vi "USB2XXX_LINEX_MasterSchTest.vi"() -> ()   [LabVIEW 2010]
panel:
  in  "Get Sch":bool
  out "设置调度表成功？":bool
  in  "pInMsg 3":T1={"Timestamp"=50, "MsgType"=2, "CheckType"=0, "DataLen"=0, "Sync"=85, "PID"=3, "Data[0]"=0, "Data[1]"=0, "Data[2]"=0, "Data[3]"=0, "Data[4]"=0, "Data[5]"=0, "Data[6]"=0, "Data[7]"=0, "Check"=0, "Reserve"=0, "Reserve"=0} {"Sync" format="%x"; "PID" format="%x"; "Data[0]" format="%x"; "Data[1]" format="%x"; "Data[2]" format="%x"; "Data[3]" format="%x"; "Data[4]" format="%x"; "Data[5]" format="%x"; "Data[6]" format="%x"; "Data[7]" format="%x"; "Check" format="%x"; "Reserve" format="%x"; "Reserve" format="%x"}
  in  "pInMsg 2":T1={"Timestamp"=50, "MsgType"=1, "CheckType"=0, "DataLen"=8, "Sync"=85, "PID"=2, "Data[0]"=17, "Data[1]"=34, "Data[2]"=51, "Data[3]"=68, "Data[4]"=85, "Data[5]"=102, "Data[6]"=119, "Data[7]"=136, "Check"=0, "Reserve"=0, "Reserve"=0} {"Sync" format="%x"; "PID" format="%x"; "Data[0]" format="%x"; "Data[1]" format="%x"; "Data[2]" format="%x"; "Data[3]" format="%x"; "Data[4]" format="%x"; "Data[5]" format="%x"; "Data[6]" format="%x"; "Data[7]" format="%x"; "Check" format="%x"; "Reserve" format="%x"; "Reserve" format="%x"}
  out "pOutMsg":T2(array[cluster]) {"Sync" format="%x"; "PID" format="%x"; "Data[0]" format="%x"; "Data[1]" format="%x"; "Data[2]" format="%x"; "Data[3]" format="%x"; "Data[4]" format="%x"; "Data[5]" format="%x"; "Data[6]" format="%x"; "Data[7]" format="%x"; "Check" format="%x"}
  in  "pInMsg":T1={"Timestamp"=50, "MsgType"=1, "CheckType"=0, "DataLen"=8, "Sync"=85, "PID"=1, "Data[0]"=1, "Data[1]"=2, "Data[2]"=3, "Data[3]"=4, "Data[4]"=5, "Data[5]"=6, "Data[6]"=7, "Data[7]"=8, "Check"=0, "Reserve"=0, "Reserve"=0} {"Sync" format="%x"; "PID" format="%x"; "Data[0]" format="%x"; "Data[1]" format="%x"; "Data[2]" format="%x"; "Data[3]" format="%x"; "Data[4]" format="%x"; "Data[5]" format="%x"; "Data[6]" format="%x"; "Data[7]" format="%x"; "Check" format="%x"; "Reserve" format="%x"; "Reserve" format="%x"}
  out "function return":i32
  in  "BaudRate":u32=9600
  in  "Channel Index":u8(ring) items=["CH0"]
  in  "Device Index":i32(ring) items=["0", "1", "2", "3", "4", "5"]
  out "Flag(T:Write;F:Read)":bool=TRUE
  in  "stop":bool
  in  "Read":bool
  in  "Write":bool
  # "点击开始后，适配器自动发送界面中的3帧数据，点击读取调度表按钮，可以获取调度表运行数据"
  # "波特率一定要设置，否则程序可能出错"
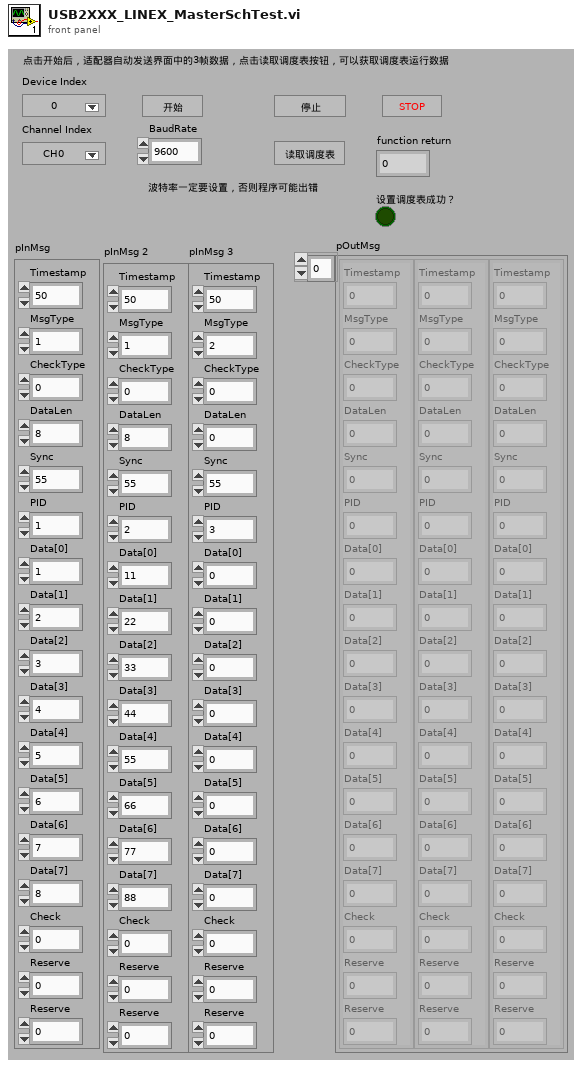
[diagram p1: front panel]
types:
  T1 = cluster{"Timestamp":u32, "MsgType":u8, "CheckType":u8, "DataLen":u8, "Sync":u8, "PID":u8, "Data[0]":u8, "Data[1]":u8, "Data[2]":u8, "Data[3]":u8, "Data[4]":u8, "Data[5]":u8, "Data[6]":u8, "Data[7]":u8, "Check":u8, "Reserve":u8, "Reserve":u8}
  T2 = cluster{"Timestamp":u32, "MsgType":u8, "CheckType":u8, "DataLen":u8, "Sync":u8, "PID":u8, "Data[0]":u8, "Data[1]":u8, "Data[2]":u8, "Data[3]":u8, "Data[4]":u8, "Data[5]":u8, "Data[6]":u8, "Data[7]":u8, "Check":u8, "Reserve":u8, "Reserve":u8}[]
  T3 = enum16{"Init", "Write", "Read", "Idel", "Close", "GetSch"}
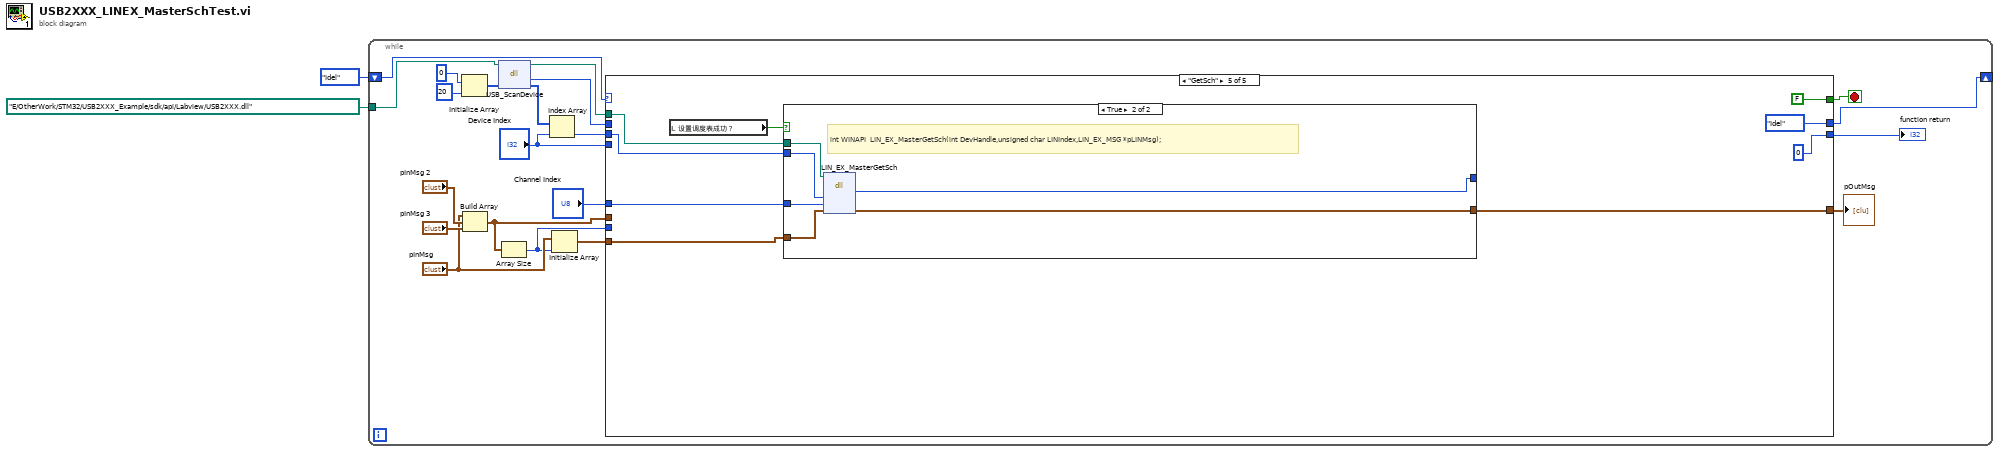
[diagram p0: block diagram]
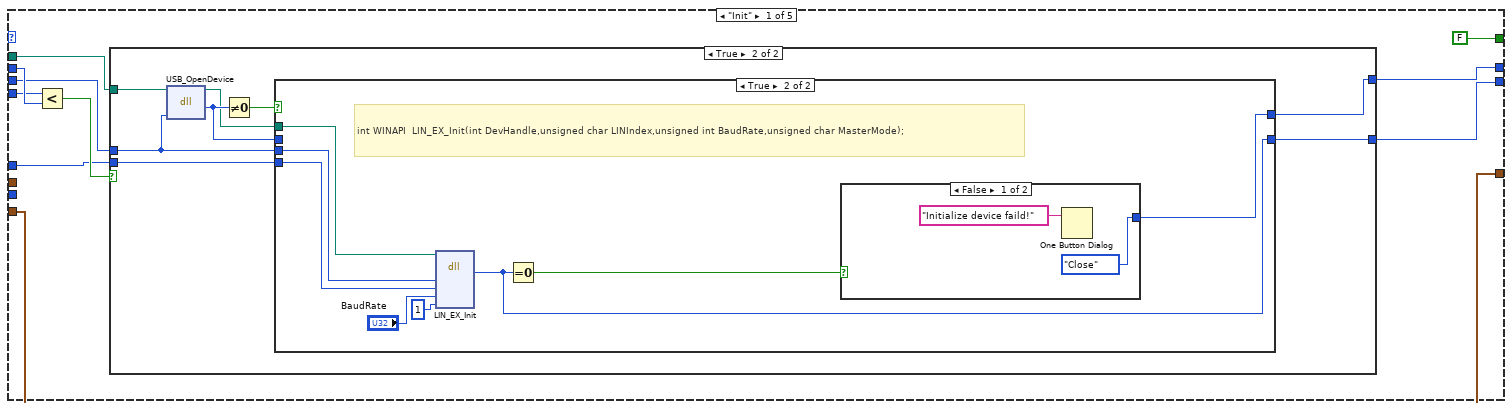
[diagram p2: hidden frame]
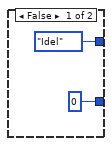
[diagram p3: hidden frame]
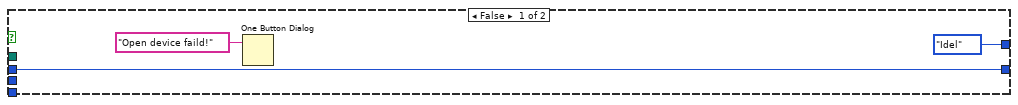
[diagram p4: hidden frame]
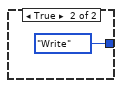
[diagram p5: hidden frame]
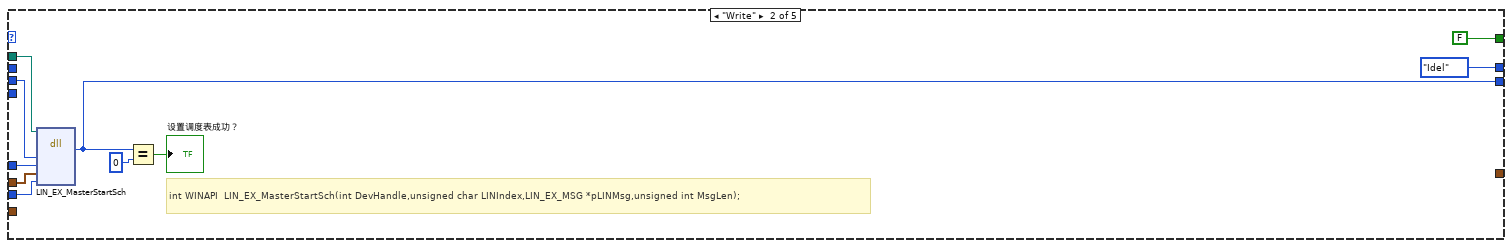
[diagram p6: hidden frame]
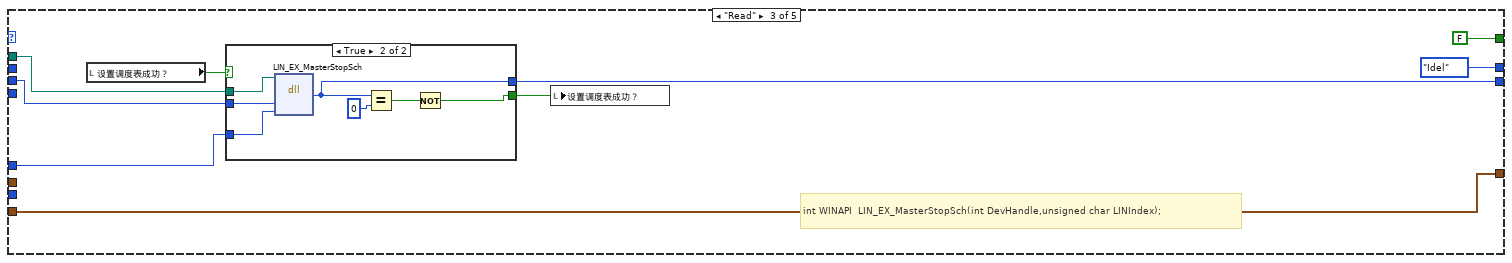
[diagram p7: hidden frame]
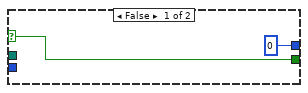
[diagram p8: hidden frame]
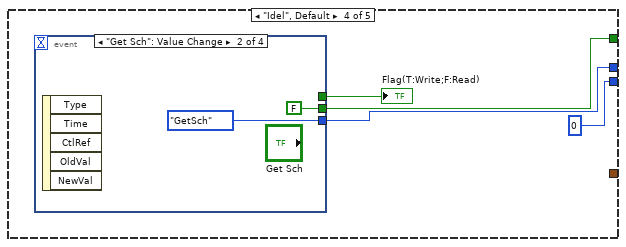
[diagram p9: hidden frame]
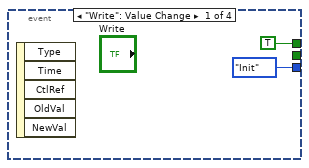
[diagram p10: hidden frame]
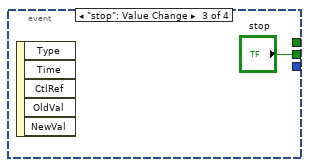
[diagram p11: hidden frame]
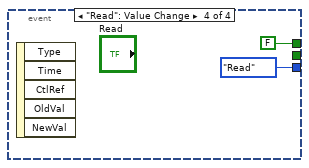
[diagram p12: hidden frame]
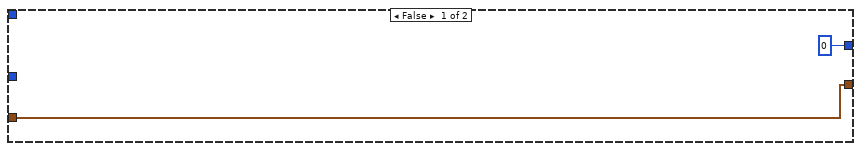
[diagram p13: hidden frame]
diagram:
  n1 = while {
    shift-right: [w22] -> _
    shift-left: T3."Idel" ("Enum") -> [w23]
    tunnel: path "E:/OtherWork/STM32/USB2XXX_Example/sdk/api/Labview/USB2XXX.dll" ("path in") -> [w4]
    stop <- w20 stop-if-true
    n2 = Initialize Array(0, 20 ("dimension size")) -> (w19:i32[])
    n3 = Build Array("pInMsg", "pInMsg 2", "pInMsg 3") -> (w6:T2)
    n4 = dll-call lib="E:/OtherWork/STM32/USB2XXX_Example/trunk/Labview/PublicFiles/USB2XXX.dll" fn="USB_ScanDevice"(path in=w4, "pDevNum"=w19) -> (path out=w3:path, "return type"=w15:i32, "pDevNum"=w16:i32[])  [unwired: 2 in, 1 out]
    n5 = Array Size(array=w6) -> (size(s)=w5:i32)
    n6 = Index Array(array=w16, index="Device Index") -> (element=w10:i32)
    n7 = Initialize Array("pInMsg", w5) -> (w13:T2)
    n8 = case shown="\"GetSch\"" w23 {
      tunnel: [w32 T3."Idel" ("Enum") T3."Idel" ("Enum") w87 T3."Idel" ("Enum")] -> w22
      tunnel: w10 -> [w28 w62 w71 _ w102]
      tunnel: "Channel Index" -> [w31 w63 w70 _ w101]
      tunnel: [FALSE FALSE FALSE w88 FALSE] -> w20
      tunnel: w15 -> [w29 _ _ _ _]
      tunnel: "Device Index" -> [w27 _ _ _ _]
      tunnel: w5 -> [_ w65 _ _ _]
      tunnel: w13 -> [w26 _ w74 _ w100]
      tunnel: w6 -> [_ w64 _ _ _]
      tunnel: [w26 _ w74 _ w99] -> w12
      tunnel: [w25 w61 w73 0 ("return type") 0 ("return type")] -> w11
      tunnel: w3 -> [w24 w58 w68 _ w97]
      frame "Init" {
        n9 = Less?(x=w27, y=w29) -> (x < y?=w33:bool)
        n10 = case shown="True" w33 {
          tunnel: w28 -> [_ w41]
          tunnel: w31 -> [_ w42]
          tunnel: [T3."Idel" ("Enum") w40] -> w32
          tunnel: [0 ("return type") w39] -> w25
          tunnel: w24 -> [_ w37]
          frame False {
          }
          frame True {
            n11 = dll-call lib="E:/OtherWork/STM32/USB2XXX_Example/trunk/Labview/PublicFiles/USB2XXX.dll" fn="USB_OpenDevice"(path in=w37, "DevIndex"=w41) -> (path out=w36:path, "return type"=w38:u8)  [unwired: 3 in, 1 out]
            n12 = Not Equal To 0?(x=w38) -> (x != 0?=w43:bool)
            n13 = case shown="True" w43 {
              tunnel: w42 -> [_ w50]
              tunnel: w41 -> [_ w51]
              tunnel: [T3."Idel" ("Enum") w53] -> w40
              tunnel: [w44 w48] -> w39
              tunnel: w38 -> [w44 _]
              tunnel: w36 -> [_ w47]
              frame False {
                n14 = One Button Dialog(message="Open device faild!") -> ()  [unwired: 1 in, 1 out]
              }
              frame True {
                # "int WINAPI  LIN_EX_Init(int DevHandle,unsigned char LINIndex,unsigned int BaudRate,unsigned char MasterMode);"
                n15 = dll-call lib="E:/OtherWork/STM32/USB2XXX_Example/trunk/Labview/PublicFiles/USB2XXX.dll" fn="LIN_EX_Init"(path in=w47, "DevHandle"=w51, "LINIndex"=w50, "BaudRate"="BaudRate", "MasterMode"=u8 1) -> ("return type"=w48:i32)  [unwired: 6 in, 2 out]
                n16 = Equal To 0?(x=w48) -> (x = 0?=w54:bool)
                n17 = case shown="False" w54 {
                  tunnel: [T3."Close" ("Enum") T3."Write" ("Enum")] -> w53
                  frame False {
                    n18 = One Button Dialog(message="Initialize device faild!") -> ()  [unwired: 1 in, 1 out]
                  }
                  frame True {
                  }
                }
              }
            }
          }
        }
      }
      frame "Write" {
        # "int WINAPI  LIN_EX_MasterStartSch(int DevHandle,unsigned char LINIndex,LIN_EX_MSG *pLINMsg,unsigned int MsgLen);"
        n19 = dll-call lib="E:/OtherWork/STM32/USB2XXX_Example/trunk/Labview/PublicFiles/USB2XXX.*" fn="LIN_EX_MasterStartSch"(path in=w58, "DevHandle"=w62, "LINIndex"=w63, "pLINMsg"=w64, "MsgLen"=w65) -> ("return type"=w61:i32)  [unwired: 6 in, 2 out]
        n20 = Equal?(x=w61, y=0) -> (x = y?=→"设置调度表成功？":bool)
      }
      frame "Read" {
        # "int WINAPI  LIN_EX_MasterStopSch(int DevHandle,unsigned char LINIndex);"
        n21 = local read "设置调度表成功？"() -> (w72:bool)
        n22 = case shown="True" w72 {
          selector: w72 -> [w77 _]
          tunnel: [0 w82] -> w73
          tunnel: [w77 w80] -> w69
          tunnel: w71 -> [_ w84]
          tunnel: w70 -> [_ w83]
          tunnel: w68 -> [_ w79]
          frame False {
          }
          frame True {
            n23 = dll-call lib="E:/OtherWork/STM32/USB2XXX_Example/trunk/Labview/PublicFiles/USB2XXX.*" fn="LIN_EX_MasterStopSch"(path in=w79, "DevHandle"=w84, "LINIndex"=w83) -> ("return type"=w82:i32)  [unwired: 4 in, 2 out]
            n24 = Equal?(x=w82, y=0) -> (x = y?=w81:bool)
            n25 = Not(x=w81) -> (.not. x?=w80:bool)
          }
        }
        n26 = local write "设置调度表成功？"(w69) -> ()
      }
      frame "Idel", Default {
        n27 = event shown="[1] \"Get Sch\": Value Change" {
          selector: _ -> [_ _ _ _]
          dyn-events: _ -> [_ _ _ _]
          timeout: _ -> [_ _ _ _]
          tunnel: [TRUE _ _ FALSE] -> w89
          tunnel: [_ FALSE ("stop") "stop" _] -> w88
          tunnel: [T3."Init" ("Enum") T3."GetSch" ("Enum") _ T3."Read" ("Enum")] -> w87
          event "Write": Value Change {
            n28 = event-data() -> ()  [unwired: 1 in, 5 out]
          }
          event "Get Sch": Value Change {
            n29 = event-data() -> ()  [unwired: 1 in, 5 out]
          }
          event "stop": Value Change {
            n30 = event-data() -> ()  [unwired: 1 in, 5 out]
          }
          event "Read": Value Change {
            n31 = event-data() -> ()  [unwired: 1 in, 5 out]
          }
        }
        "Flag(T:Write;F:Read)" <- w89
      }
      frame "GetSch" {
        n32 = local read "设置调度表成功？"() -> (w103:bool)
        n33 = case shown="True" w103 {
          tunnel: w102 -> [_ w113]
          tunnel: w101 -> [_ w112]
          tunnel: w100 -> [w107 w111]
          tunnel: [0 w110] -> _
          tunnel: [w107 w109] -> w99
          tunnel: w97 -> [_ w108]
          frame False {
          }
          frame True {
            # "int WINAPI  LIN_EX_MasterGetSch(int DevHandle,unsigned char LINIndex,LIN_EX_MSG *pLINMsg);"
            n34 = dll-call lib="E:/OtherWork/STM32/USB2XXX_Example/trunk/Labview/PublicFiles/USB2XXX.*" fn="LIN_EX_MasterGetSch"(path in=w108, "DevHandle"=w113, "LINIndex"=w112, "pLINMsg"=w111) -> ("return type"=w110:i32, "pLINMsg"=w109:T2)  [unwired: 4 in, 2 out]
          }
        }
      }
    }
    "pOutMsg" <- w12
    "function return" <- w11
  }
